vi "TestStand, Table to TS_Result.vi"(6 "row (0)":i32, 8 "error in":errorcluster, 11 "Tbl Refnum":refnum<vi>) -> (0 "error out":errorcluster, 2 "TestStand Result":T1={"Measurement Name"="", "Result"=nan, "Low Limit"=nan, "High Limit"=nan, "Units"="", "Comp"="", "DataFmt"="", "LimitFmt"=""} {"Result" format="%.3g"; "High Limit" format="%.3g"; "Low Limit" format="%.3g"}, 3 "Tbl Refnum out":refnum<vi>)   [LabVIEW 2010]
doc: "Converts one row from a Test Criteria Table to a TestStand Result cluster."
uses:
  TestStand_Result Control.ctl
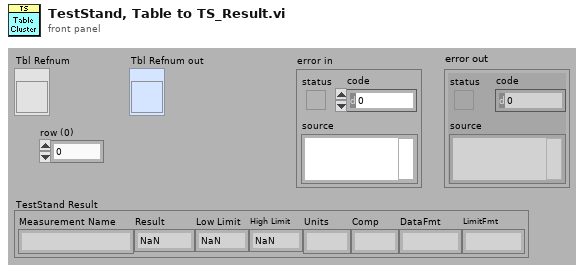
[diagram p1: front panel]
types:
  T1 = typedef "TestStand_Result Control.ctl" = cluster{"Measurement Name":string, "Result":dbl, "Low Limit":dbl, "High Limit":dbl, "Units":string, "Comp":string, "DataFmt":string, "LimitFmt":string}
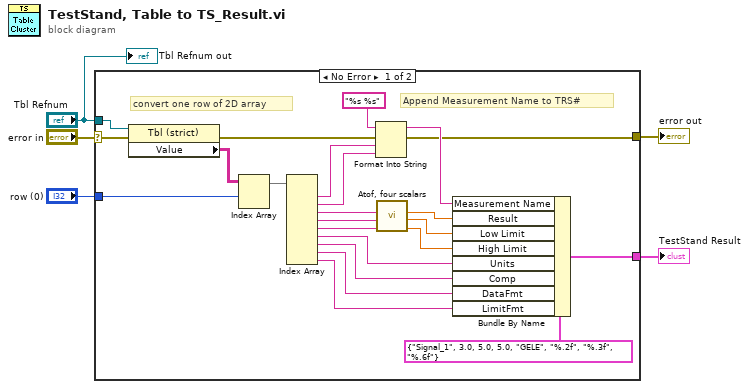
[diagram p0: block diagram]
diagram:
  n1 = case shown="No Error" "error in" {
    selector: "error in" -> [w26 w29]
    tunnel: "Tbl Refnum" -> [w28 _]
    tunnel: [w27 _] -> w1
    tunnel: [w6 w29] -> w5
    tunnel: "row (0)" -> [w24 _]
    frame No Error {
      # "Append Measurement Name to TRS#"
      # "convert one row of 2D array"
      n2 = property class="Tbl (strict)"(reference=w28, error in=w26) -> (error out=w7:errorcluster, "Value"=w23:string[][])  [unwired: 1 out]
      n3 = Index Array(array=w23, index (row)=w24) -> (element=w22:string[])  [unwired: 1 in]
      n4 = Index Array(array=w22) -> (element #1=w9:string, element #2=w10:string, element #3=w15:string, element #4=w16:string, element #5=w17:string, element #6=w18:string, element #7=w19:string, element #8=w20:string, element #9=w21:string)  [unwired: 9 in]
      n5 = Format Into String(format string="%s %s", error in=w7, w9, w10) -> (resulting string=w8:string, error out=w6:errorcluster)  [unwired: 1 in]
      n6 = call "Atof, four scalars.vi"("string 4"=w17, "string 3"=w16, "string 2"=w15) -> ("number 4"=w14:dbl, "number 3"=w13:dbl, "number 2"=w12:dbl)  [unwired: 1 in, 1 out]
      n7 = Bundle By Name(cluster=T1 {"Measurement Name"="Signal_1", "Result"=3.0, "Low Limit"=5.0, "High Limit"=5.0, "Units"="GELE", "Comp"="%.2f", "DataFmt"="%.3f", "LimitFmt"="%.6f"} ("TS_Result"), "Measurement Name"=w8, "Result"=w12, "Low Limit"=w13, "High Limit"=w14, "Units"=w18, "Comp"=w19, "DataFmt"=w20, "LimitFmt"=w21) -> (w27:T1)
    }
    frame Error {
    }
  }
  "error out" <- w5
  "TestStand Result" <- w1
  "Tbl Refnum out" <- "Tbl Refnum"
